vi "Update_Ch_Names.vi"(1 "Ch Name in":string[](array[string])) -> (0 "Ch Name Out":string[](array[string]))   [LabVIEW 2010]
uses:
  Globals/Meas_global.vi
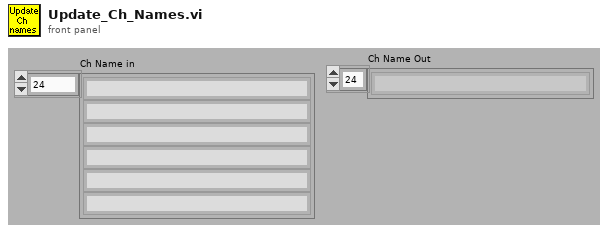
[diagram p1: front panel]
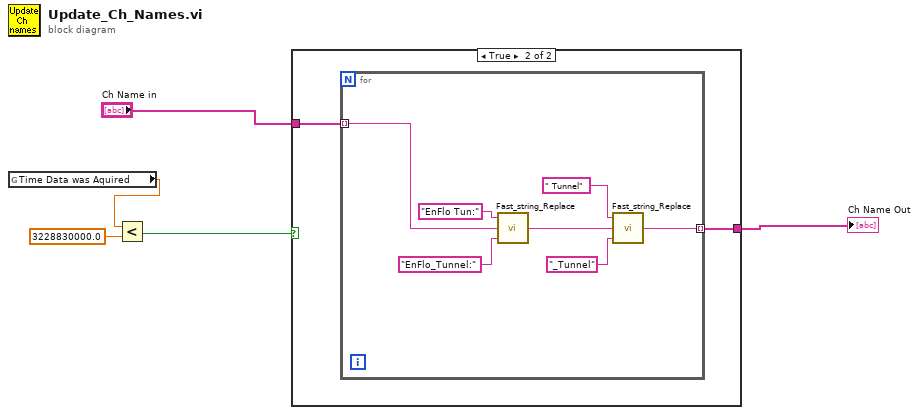
[diagram p0: block diagram]
diagram:
  n1 = global read "Meas_global.vi" "Time Data was Aquired"() -> (w3:dbl)
  n2 = Less?(x=w3, y=3228830000.0) -> (x < y?=w1:bool)
  n3 = case shown="True" w1 {
    tunnel: "Ch Name in" -> [w6 w8]
    tunnel: [w6 w7] -> w4
    frame False {
    }
    frame True {
      n4 = for {
        tunnel: w8 -> [w14] mode=indexing
        tunnel: [w10] -> w7 mode=indexing
        n5 = call "Fast_string_Replace.vi"("Replace match with:"="EnFlo_Tunnel:" ("regular expression"), "Input String"=w14, "regular expression"="EnFlo Tun:") -> ("Output String"=w9:string)  [unwired: 2 out]
        n6 = call "Fast_string_Replace.vi"("Replace match with:"="_Tunnel" ("regular expression"), "Input String"=w9, "regular expression"=" Tunnel") -> ("Output String"=w10:string)  [unwired: 2 out]
      }
    }
  }
  "Ch Name Out" <- w4
